vi "LesenUndSchreiben(SubVI).vi"(0 "Score":T1, 1 "file path (dialog if empty)":path caption="Dateipfad (Dialog, wenn leer)", 5 "Score 2":T1, 7 "Score 3":T1, 9 "Score 4":T1, 12 "gameOver":bool, 15 "resetOut":bool) -> (4 "Score 5":T1, 6 "Score 6":T1, 8 "Score 7":T1, 10 "Score 8":T1)   [LabVIEW 2017]
uses:
  <vilib>/Utility/file.llb/Write Delimited Spreadsheet (DBL).vi
  <vilib>/Utility/file.llb/Read Delimited Spreadsheet (I64).vi
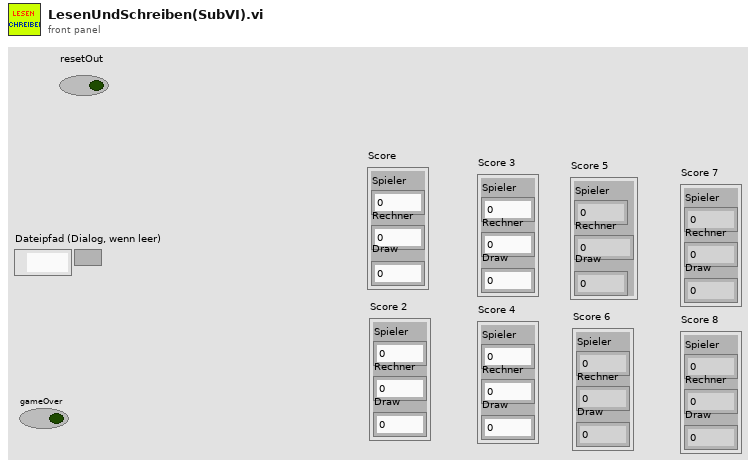
[diagram p1: front panel]
types:
  T1 = cluster{"Spieler":dbl, "Rechner":dbl, "Draw":dbl}
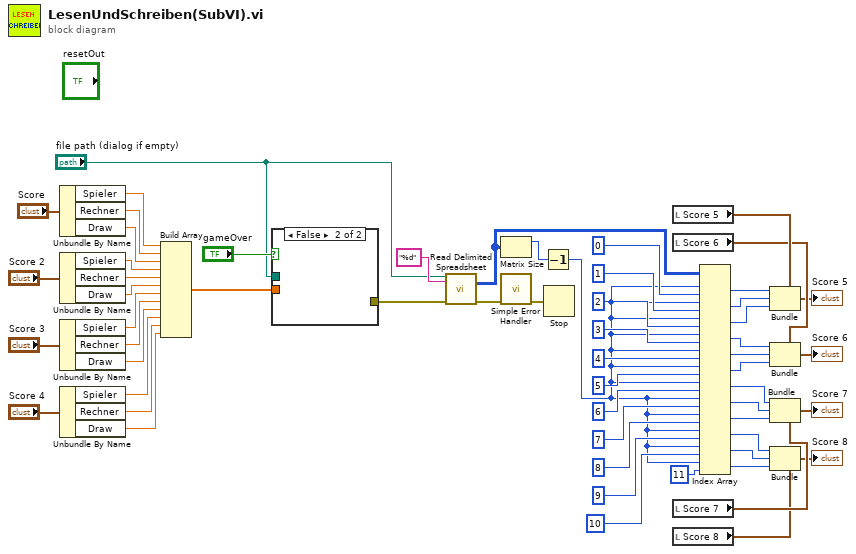
[diagram p0: block diagram]
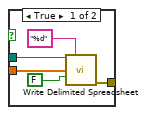
[diagram p2: hidden frame]
diagram:
  n1 = Unbundle By Name("Score") -> ("Spieler"=w55:dbl, "Rechner"=w54:dbl, "Draw"=w53:dbl)
  n2 = Unbundle By Name("Score 2") -> ("Spieler"=w47:dbl, "Rechner"=w46:dbl, "Draw"=w45:dbl)
  n3 = Unbundle By Name("Score 3") -> ("Spieler"=w44:dbl, "Rechner"=w43:dbl, "Draw"=w42:dbl)
  n4 = Unbundle By Name("Score 4") -> ("Spieler"=w41:dbl, "Rechner"=w40:dbl, "Draw"=w39:dbl)
  n5 = Build Array(w55, w54, w53, w47, w46, w45, w44, w43, w42, w41, w40, w39) -> (w1:dbl[])
  n6 = case shown="False" "gameOver" {
    tunnel: "file path (dialog if empty)" -> [w61 _]
    tunnel: [w60 _] -> w37
    tunnel: w1 -> [w59 _]
    frame True {
      n7 = call-poly <vilib>:"Write Delimited Spreadsheet.vi"("file path (dialog if empty)"=w61, "format (%.3f)"="%d" ("format (%s)"), "1D data"=w59, "append to file? (new file:F)"=FALSE) -> ("error out"=w60:errorcluster)  [unwired: 10 in, 1 out]
    }
    frame False {
    }
  }
  n8 = call-poly <vilib>:"Read Delimited Spreadsheet.vi"("file path (dialog if empty)"="file path (dialog if empty)", "format (%d)"="%d" ("format (%s)"), "error in (no error)"=w37) -> ("all rows"=w36:i64[][], "error out"=w56:errorcluster)  [unwired: 7 in, 4 out]
  n9 = Matrix Size(0:w36) -> (1:w6:i32)  [unwired: 1 out]
  n10 = call <vilib>:"Simple Error Handler.vi"("error in (no error)"=w56) -> ("error out"=w58:errorcluster)  [unwired: 4 in, 4 out]
  n11 = Decrement(x=w6) -> (x-1=w5:i32)
  n12 = Stop(stop? (T)=w58) -> ()
  n13 = local read "Score 5"() -> (w35:T1)
  n14 = local read "Score 6"() -> (w34:T1)
  n15 = local read "Score 7"() -> (w33:T1)
  n16 = local read "Score 8"() -> (w32:T1)
  n17 = Index Array(array=w36, index (row) #1=w5, index (col) #1=0 ("Deaktivierter Index (Spalte)"), index (row) #2=w5, index (col) #2=1 ("Deaktivierter Index (Spalte)"), index (row) #3=w5, index (col) #3=2 ("Deaktivierter Index (Spalte)"), index (row) #4=w5, index (col) #4=3 ("Deaktivierter Index (Spalte)"), index (row) #5=w5, index (col) #5=4 ("Deaktivierter Index (Spalte)"), index (row) #6=w5, index (col) #6=5 ("Deaktivierter Index (Spalte)"), index (row) #7=w5, index (col) #7=6 ("Deaktivierter Index (Spalte)"), index (row) #8=w5, index (col) #8=7 ("Deaktivierter Index (Spalte)"), index (row) #9=w5, index (col) #9=8 ("Deaktivierter Index (Spalte)"), index (row) #10=w5, index (col) #10=9 ("Deaktivierter Index (Spalte)"), index (row) #11=w5, index (col) #11=10 ("Deaktivierter Index (Spalte)"), index (row) #12=w5, index (col) #12=11 ("Deaktivierter Index (Spalte)")) -> (element #1=w30:i64, element #2=w29:i64, element #3=w28:i64, element #4=w27:i64, element #5=w26:i64, element #6=w25:i64, element #7=w24:i64, element #8=w23:i64, element #9=w22:i64, element #10=w21:i64, element #11=w20:i64, element #12=w19:i64)
  n18 = Bundle(cluster=w35, "Spieler"=w30, "Rechner"=w29, "Draw"=w28) -> (→"Score 5":T1)
  n19 = Bundle(cluster=w34, "Spieler"=w27, "Rechner"=w26, "Draw"=w25) -> (→"Score 6":T1)
  n20 = Bundle(cluster=w33, "Spieler"=w24, "Rechner"=w23, "Draw"=w22) -> (→"Score 7":T1)
  n21 = Bundle(cluster=w32, "Spieler"=w21, "Rechner"=w20, "Draw"=w19) -> (→"Score 8":T1)
